vi "test starburst double complete rainbow.vi"() -> ()   [LabVIEW 2015]
uses:
  connection/connection maintainer.lvclass
  client/connection client.lvclass/connection client.ctl
  message/communicator message.lvclass
  starburst/starburst.lvclass
  communicator/communicator.lvclass/communicator.ctl
  message/communicator message.lvclass/communicator message.ctl
  communicator/enqueue variety.ctl
  client/prepare client.vi
  server/prepare server.vi
  TCP client/TCP client.lvclass
  TCP/TCP server.lvclass
  Queue Client/Queue client.lvclass
  communicator/communicator.lvclass
  <vilib>/ptbypt/NI_PtbyPt.lvlib
  manager/queue manager.lvclass
  Queue server/Queue server.lvclass
panel:
  out "ClienQ 2":refnum<class "connection maintainer.lvclass">
  out "Numeric 3":dbl
  out "ClienT 2":timestamp
  out "data 2":variant
  out "ID 2":string
  in  "remake c 2":bool
  in  "c2":cluster{"ID":string, "data":string}
  in  "C to S 2":bool
  out "Numeric 2":dbl
  out "data 3":variant
  out "ID 3":string
  out "data":variant
  out "ID":string
  out "Numeric":dbl
  in  "Boolean":bool
  in  "remake c":bool
  in  "s":cluster{"ID":string, "data":string}
  in  "c1":cluster{"ID":string, "data":string}
  in  "S to C":bool
  in  "C to S":bool
  in  "exits":bool
  out "ClienT":timestamp
  out "servT":timestamp
  out "ClienQ":refnum<class "connection maintainer.lvclass">
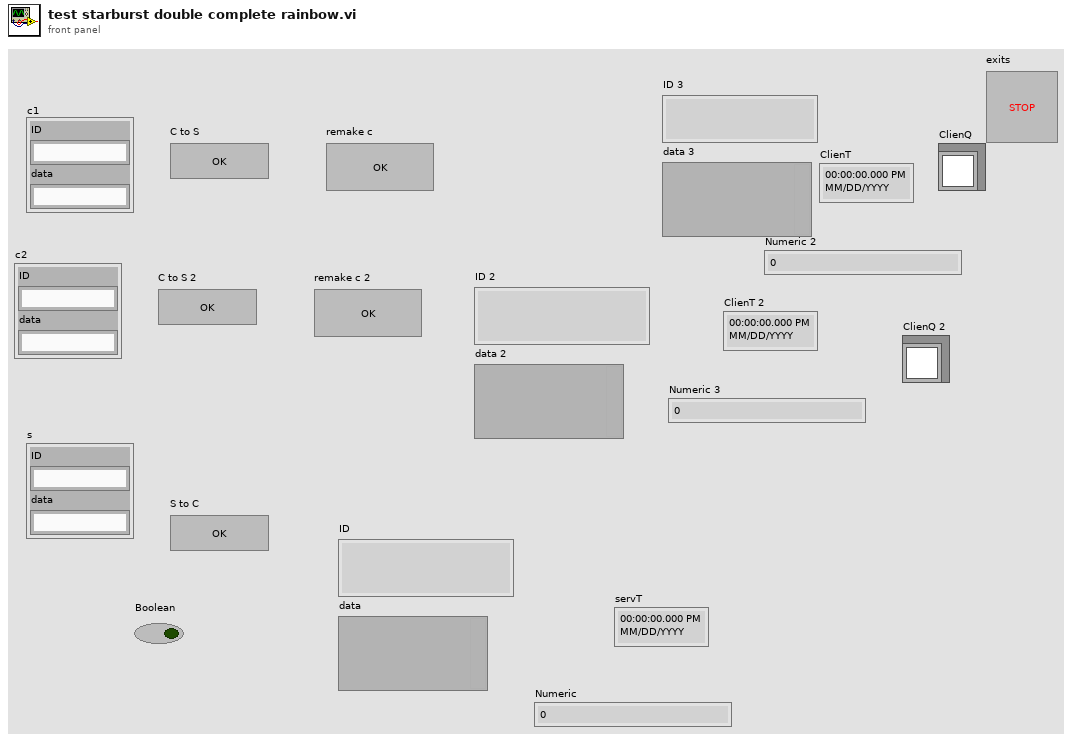
[diagram p1: front panel]
types:
  T1 = typedef "communicator.lvclass/enqueue variety.ctl" = enum16{"normal", "lossy", "priority"}
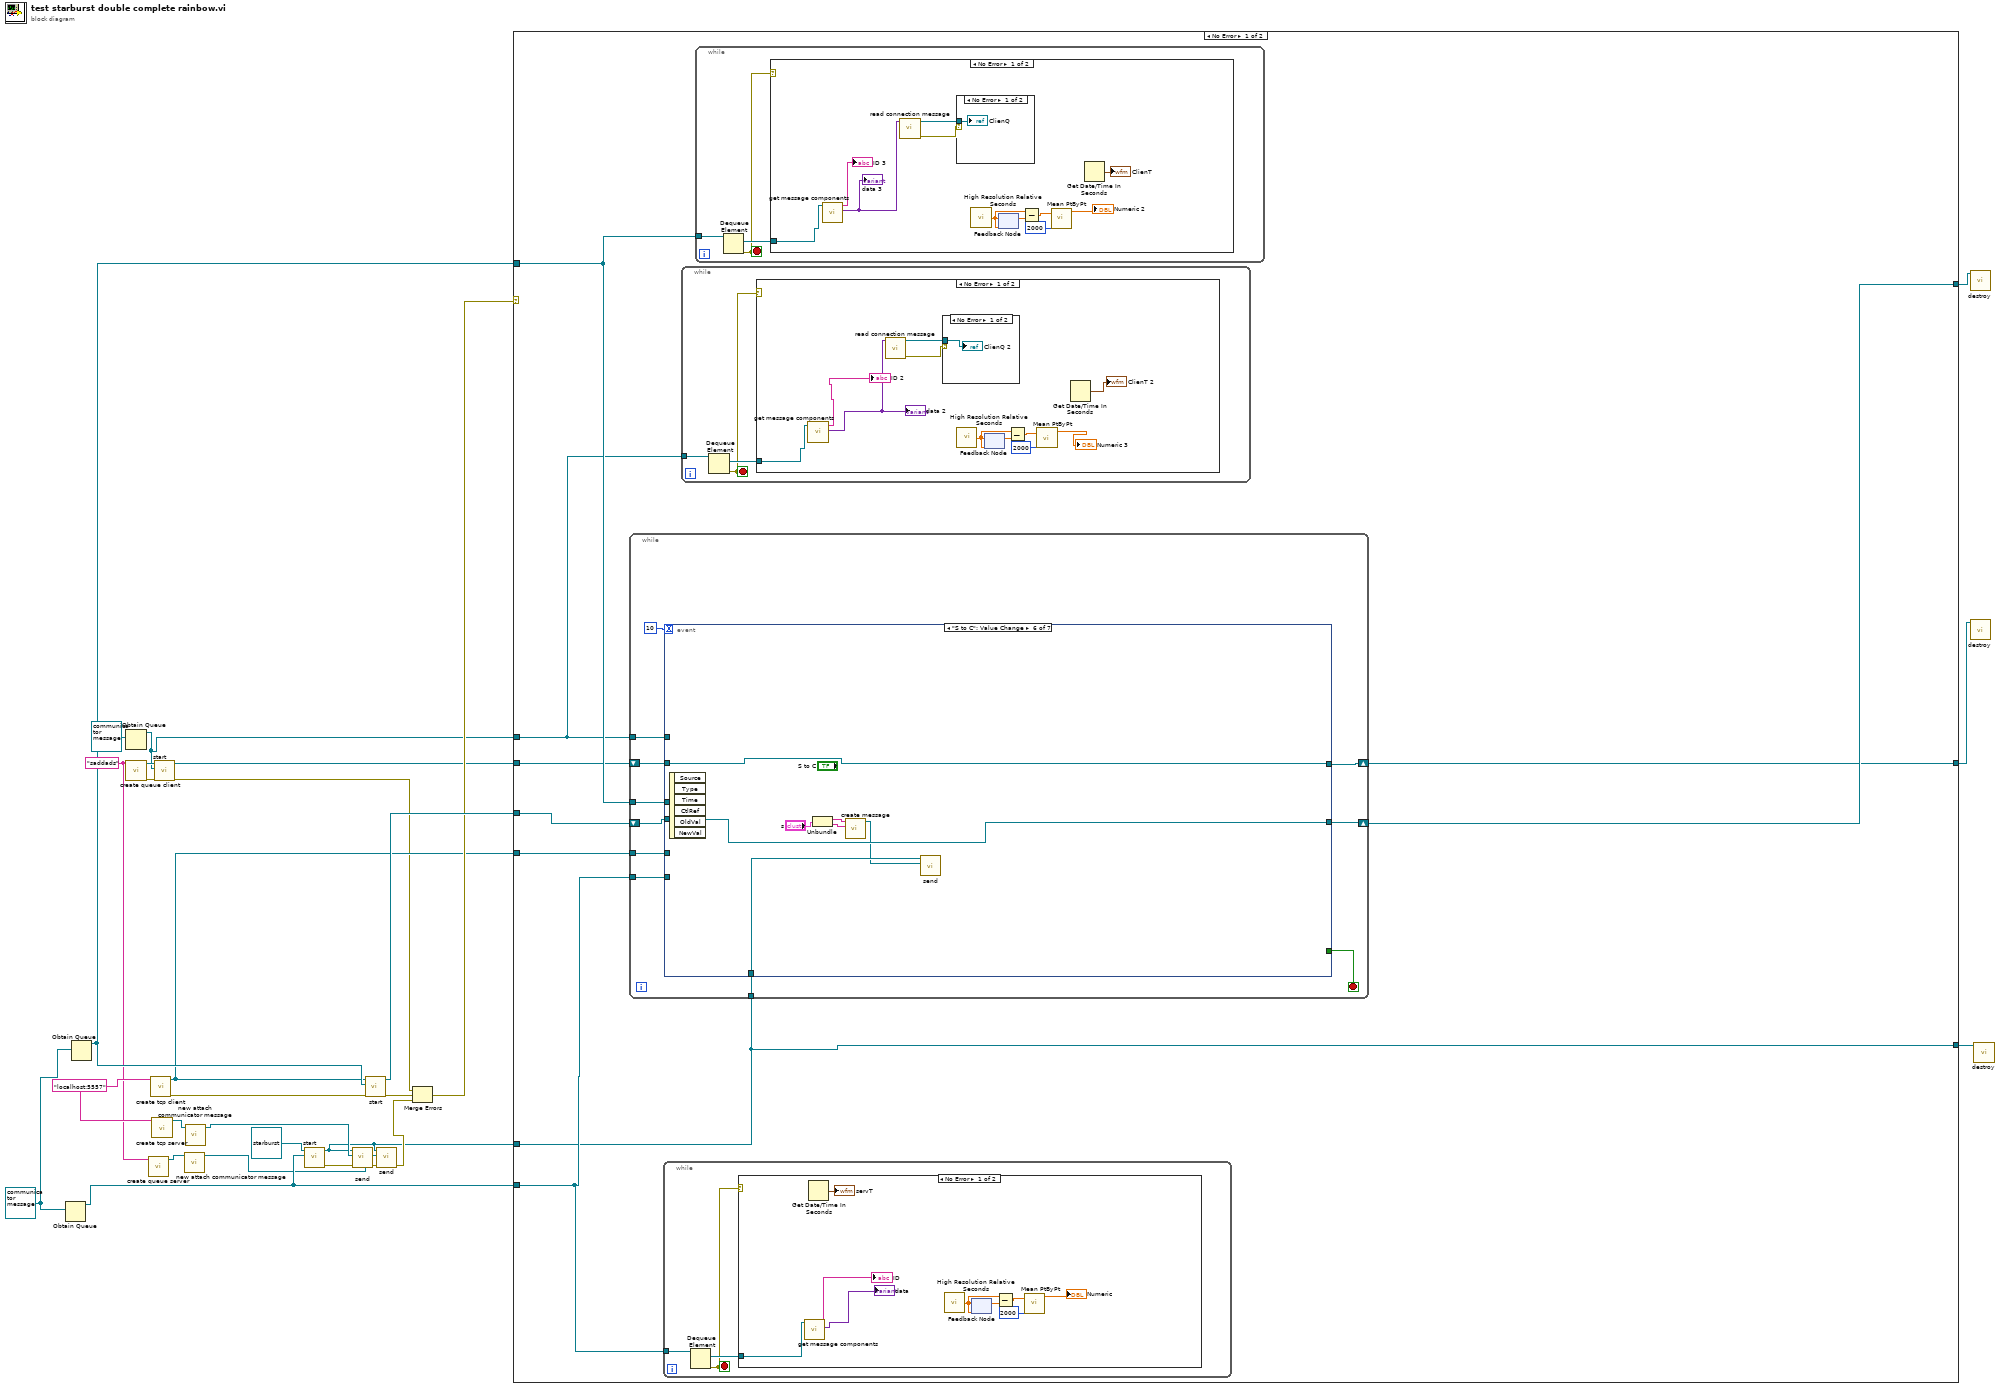
[diagram p0: block diagram]
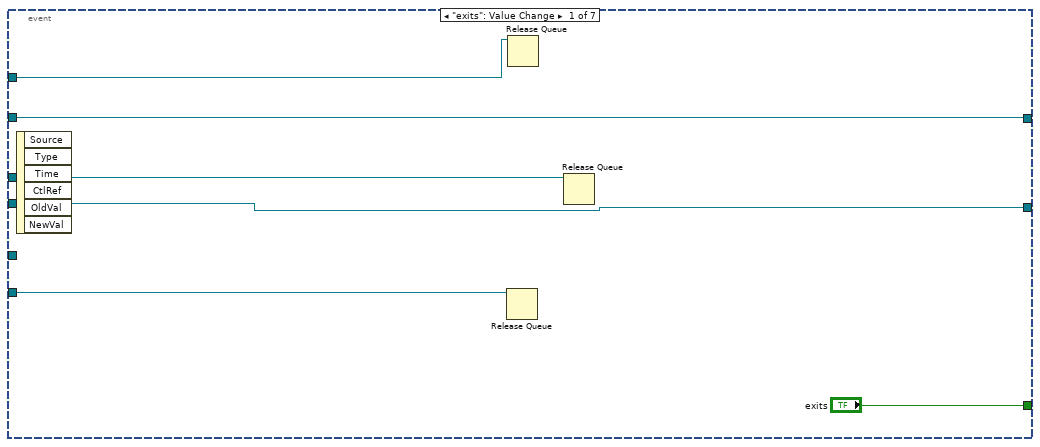
[diagram p4: hidden frame]
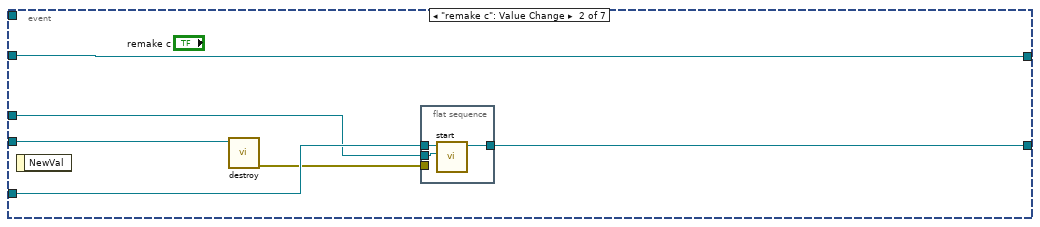
[diagram p5: hidden frame]
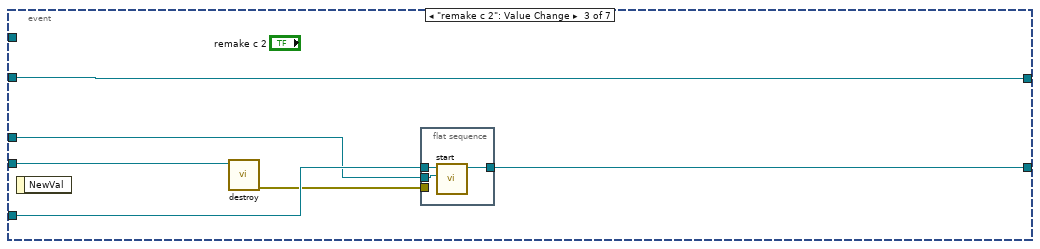
[diagram p6: hidden frame]
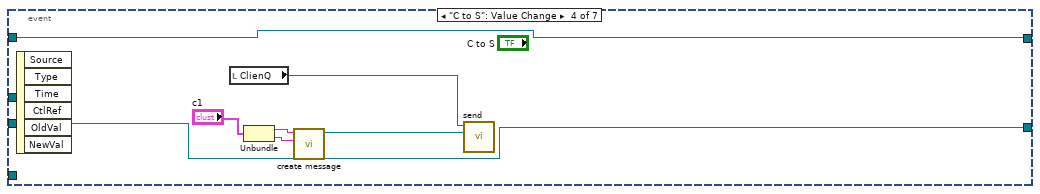
[diagram p7: hidden frame]
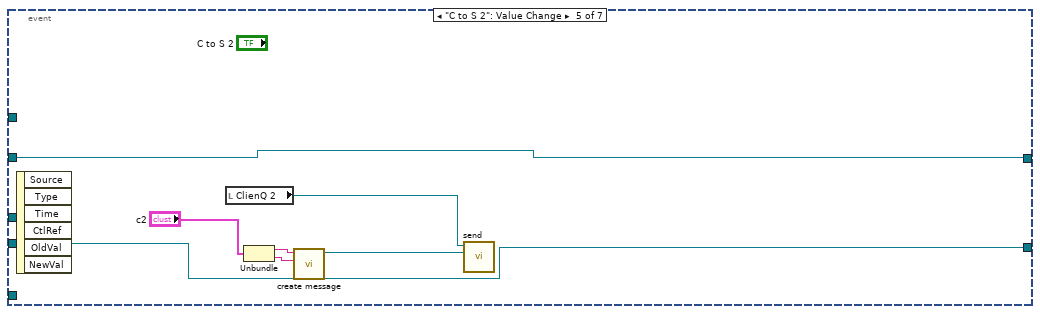
[diagram p8: hidden frame]
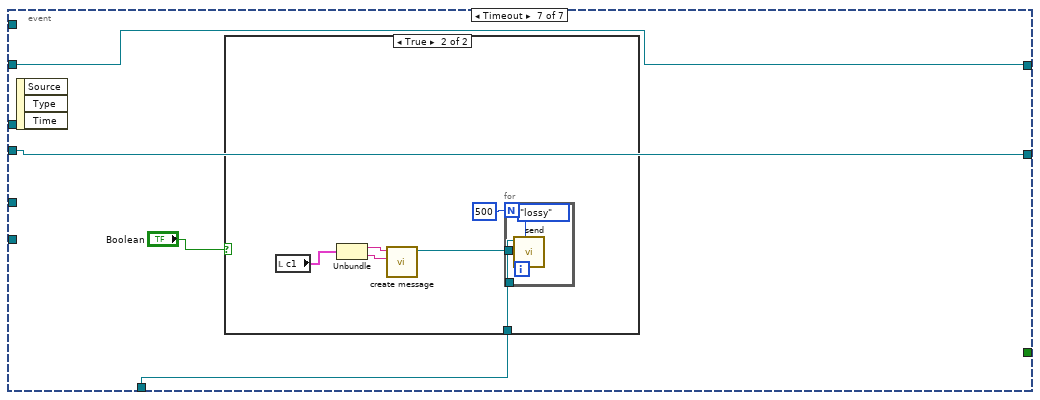
[diagram p9: hidden frame]
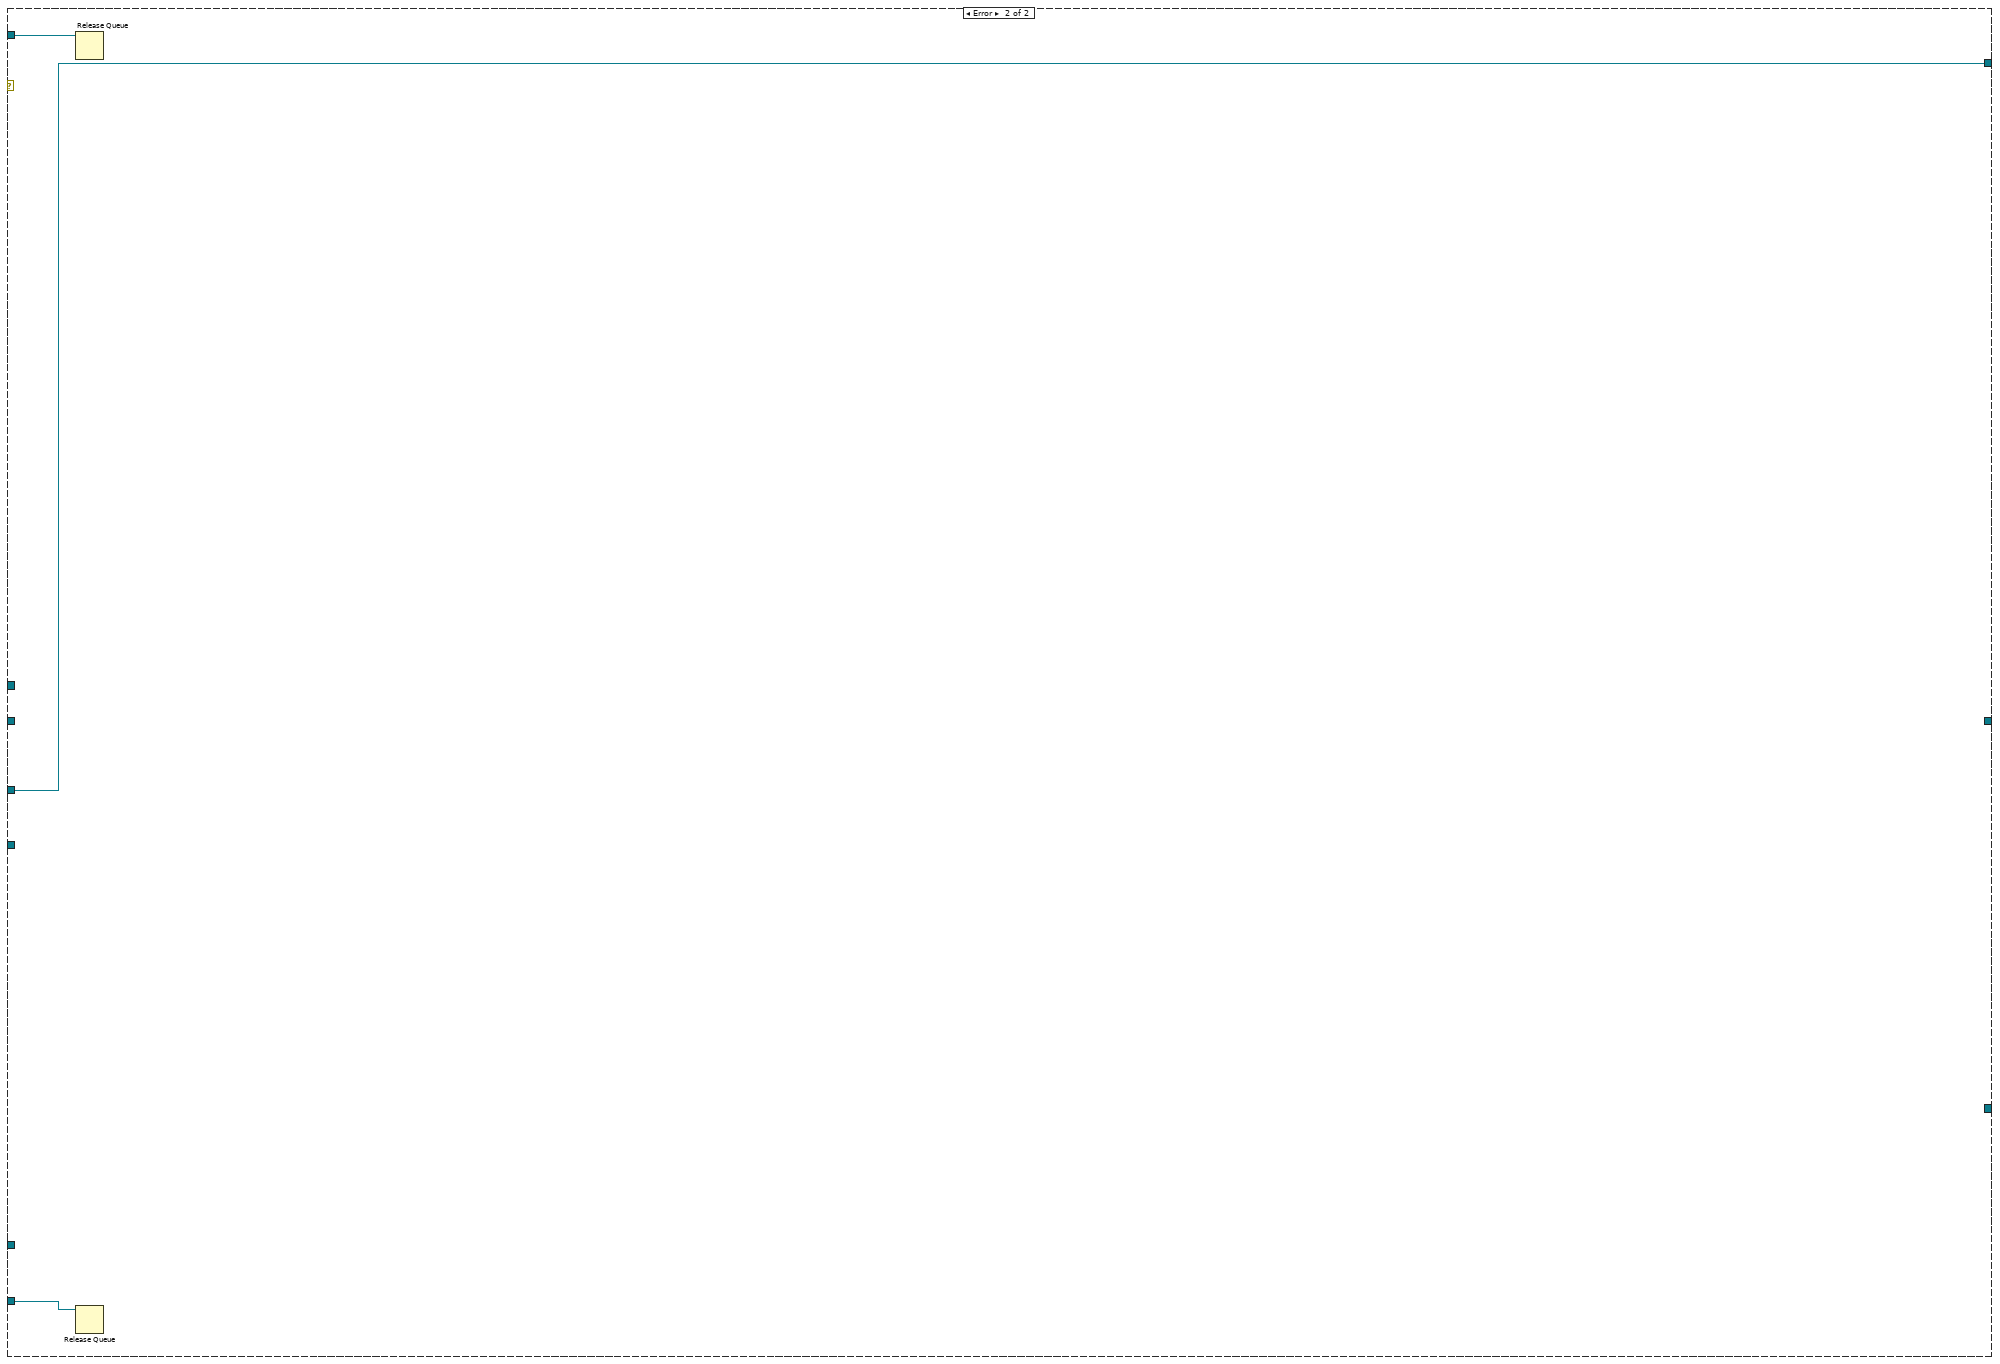
[diagram p14: hidden frame]
diagram:
  w1 = "saddads" ("connection string")
  w20 = refnum<class "communicator message.lvclass"> refnum ("message")
  w24 = "localhost:5557" ("connection string")
  n1 = Obtain Queue(element data type=w20) -> (queue out=w18:refnum<queue>)  [unwired: 4 in, 2 out]
  n2 = Obtain Queue(element data type=w20) -> (queue out=w22:refnum<queue>)  [unwired: 4 in, 2 out]
  n3 = Obtain Queue(element data type=refnum<class "communicator message.lvclass"> refnum ("communicator message.lvclass")) -> (queue out=w3:refnum<queue>)  [unwired: 4 in, 2 out]
  n4 = call "create queue client.vi"("conn string"=w1) -> ("error out"=w6:errorcluster, "TCP client out"=w7:refnum<class "Queue client.lvclass">)  [unwired: 9 in]
  n5 = call "create queue server.vi"("conn string"=w1) -> ("TCP server out"=w12:refnum<class "Queue server.lvclass">)  [unwired: 9 in, 1 out]
  n6 = call "create tcp client.vi"("conn string"=w24) -> ("error out"=w27:errorcluster, "TCP client out"=w21:refnum<class "TCP client.lvclass">)  [unwired: 9 in]
  n7 = call "create tcp server.vi"("conn string"=w24) -> ("TCP server out"=w16:refnum<class "TCP server.lvclass">)  [unwired: 9 in, 1 out]
  n8 = call-dynamic "start.vi"("error in"=w6, "queue to parent"=w3, "communicator in"=w7) -> ("error out"=w5:errorcluster, "communicator out"=w4:refnum<class "Queue client.lvclass">)  [unwired: 7 in]
  n9 = call "new attach communicator message.vi"("comm"=w12) -> ("message"=w9:refnum<class "communicator message.lvclass">)  [unwired: 9 in, 1 out]
  n10 = call "new attach communicator message.vi"("comm"=w16) -> ("message"=w14:refnum<class "communicator message.lvclass">)  [unwired: 9 in, 1 out]
  n11 = call-dynamic "start.vi"("queue to parent"=w18, "communicator in"=refnum<class "starburst.lvclass"> refnum ("starburst")) -> ("error out"=w17:errorcluster, "communicator out"=w10:refnum<class "starburst.lvclass">)  [unwired: 8 in]
  n12 = call "send.vi"("error in"=w17, "element"=w14, "communicator in"=w10) -> ("error out"=w15:errorcluster)  [unwired: 8 in]
  n13 = call-dynamic "start.vi"("error in"=w27, "queue to parent"=w22, "communicator in"=w21) -> ("error out"=w25:errorcluster, "communicator out"=w26:refnum<class "TCP client.lvclass">)  [unwired: 7 in]
  n14 = call "send.vi"("error in"=w15, "element"=w9, "communicator in"=w10) -> ("error out"=w11:errorcluster)  [unwired: 8 in]
  n15 = Merge Errors(w5, w25, w11) -> (w23:errorcluster)
  n16 = case shown="No Error" w23 {
    tunnel: [w33 w150] -> w28
    tunnel: w22 -> [w36 w151]
    tunnel: w26 -> [w35 w150]
    tunnel: w18 -> [w37 w149]
    tunnel: w21 -> [w34 _]
    tunnel: w10 -> [w32 _]
    tunnel: [w32 _] -> w13
    tunnel: w4 -> [w31 _]
    tunnel: w3 -> [w30 _]
    tunnel: [w29 _] -> w2
    frame No Error {
      n17 = while {
        tunnel: w37 -> [w62]
        tunnel: w36 -> [w61]
        tunnel: w34 -> [w59]
        shift-right: [w58] -> w33
        shift-left: w35 -> [w60]
        tunnel: w32 -> [w56]
        shift-right: [w53] -> w29
        shift-left: w31 -> [w55]
        tunnel: w30 -> [w54]
        stop <- w63 stop-if-true
        n18 = event shown="[5] \"S to C\": Value Change" {
          selector: _ -> [_ _ _ _ _ _ _]
          dyn-events: _ -> [_ _ _ _ _ _ _]
          timeout: 10 -> [_ _ _ _ _ _ _]
          tunnel: ["exits" _ _ _ _ _ _] -> w63
          tunnel: w62 -> [w68 _ _ _ _ _ _]
          tunnel: w61 -> [w67 w72 w81 _ _ _ _]
          tunnel: w60 -> [w66 w75 w84 w92 w99 w108 w112]
          tunnel: w59 -> [_ w74 w83 _ _ _ _]
          tunnel: [w66 w71 w80 w92 w99 w108 w112] -> w58
          tunnel: w56 -> [_ _ _ _ _ w104 w110]
          tunnel: w55 -> [w65 w70 w79 w88 w96 w102 w109]
          tunnel: w54 -> [w64 _ _ _ _ _ _]
          tunnel: [w65 w70 w79 w88 w96 w102 w109] -> w53
          event "exits": Value Change {
            n19 = event-data() -> ()  [unwired: 1 in, 6 out]
            n20 = Release Queue(queue=w68) -> ()  [unwired: 2 in, 3 out]
            n21 = Release Queue(queue=w64) -> ()  [unwired: 2 in, 3 out]
            n22 = Release Queue(queue=w67) -> ()  [unwired: 2 in, 3 out]
          }
          event "remake c": Value Change {
            n23 = event-data() -> ()  [unwired: 1 in, 1 out]
            n24 = call-dynamic "destroy.vi"("communicator in"=w75) -> ("error out"=w73:errorcluster)  [unwired: 10 in]
            n25 = flat-sequence {
              tunnel: w74 -> [w78]
              tunnel: w73 -> [_]
              tunnel: w72 -> [w77]
              tunnel: [w76] -> w71
              frame #0 {
                n26 = call-dynamic "start.vi"("queue to parent"=w77, "communicator in"=w78) -> ("communicator out"=w76:refnum<class "TCP client.lvclass">)  [unwired: 8 in, 1 out]
              }
            }
          }
          event "remake c 2": Value Change {
            n27 = event-data() -> ()  [unwired: 1 in, 1 out]
            n28 = call-dynamic "destroy.vi"("communicator in"=w84) -> ("error out"=w82:errorcluster)  [unwired: 10 in]
            n29 = flat-sequence {
              tunnel: w83 -> [w87]
              tunnel: w82 -> [_]
              tunnel: w81 -> [w86]
              tunnel: [w85] -> w80
              frame #0 {
                n30 = call-dynamic "start.vi"("queue to parent"=w86, "communicator in"=w87) -> ("communicator out"=w85:refnum<class "TCP client.lvclass">)  [unwired: 8 in, 1 out]
              }
            }
          }
          event "C to S": Value Change {
            n31 = event-data() -> ()  [unwired: 1 in, 6 out]
            n32 = local read "ClienQ"() -> (w94:refnum<class "connection maintainer.lvclass">)
            n33 = Unbundle("c1") -> ("ID"=w91:string, "data"=w90:string)
            n34 = call "create message.vi"("data"=w90, "ID"=w91) -> ("message"=w93:refnum<class "communicator message.lvclass">)  [unwired: 9 in]
            n35 = call "send.vi"("element"=w93, "communicator in"=w94) -> ()  [unwired: 9 in, 1 out]
          }
          event "C to S 2": Value Change {
            n36 = event-data() -> ()  [unwired: 1 in, 6 out]
            n37 = local read "ClienQ 2"() -> (w101:refnum<class "connection maintainer.lvclass">)
            n38 = Unbundle("c2") -> ("ID"=w98:string, "data"=w97:string)
            n39 = call "create message.vi"("data"=w97, "ID"=w98) -> ("message"=w100:refnum<class "communicator message.lvclass">)  [unwired: 9 in]
            n40 = call "send.vi"("element"=w100, "communicator in"=w101) -> ()  [unwired: 9 in, 1 out]
          }
          event "S to C": Value Change {
            n41 = event-data() -> ()  [unwired: 1 in, 6 out]
            n42 = Unbundle("s") -> ("ID"=w107:string, "data"=w106:string)
            n43 = call "create message.vi"("data"=w106, "ID"=w107) -> ("message"=w103:refnum<class "communicator message.lvclass">)  [unwired: 9 in]
            n44 = call "send.vi"("element"=w103, "communicator in"=w104) -> ()  [unwired: 9 in, 1 out]
          }
          event Timeout {
            n45 = event-data() -> ()  [unwired: 1 in, 3 out]
            n46 = case shown="True" "Boolean" {
              tunnel: w110 -> [_ w114]
              frame False {
              }
              frame True {
                n47 = local read "c1"() -> (w116:cluster{"ID":string, "data":string})
                n48 = Unbundle(w116) -> ("ID"=w118:string, "data"=w117:string)
                n49 = call "create message.vi"("data"=w117, "ID"=w118) -> ("message"=w115:refnum<class "communicator message.lvclass">)  [unwired: 9 in]
                n50 = for {
                  N: 500 -> [_]
                  tunnel: w115 -> [w121]
                  tunnel: w114 -> [w120]
                  n51 = call "send.vi"("enqueue setting"=enqueue_variety."lossy", "element"=w121, "communicator in"=w120) -> ()  [unwired: 8 in, 1 out]
                }
              }
            }
          }
        }
      }
      n52 = while {
        tunnel: w37 -> [w124]
        stop <- w122 stop-if-true
        n53 = Dequeue Element(queue=w124) -> (element=w123:refnum<class "communicator message.lvclass">, error out=w122:errorcluster)  [unwired: 2 in, 2 out]
        n54 = case shown="No Error" w122 {
          tunnel: w123 -> [w125 _]
          frame No Error {
            n55 = call "get message components.vi"("message"=w125) -> ("data"=→"data":variant, "ID"=→"ID":string)  [unwired: 9 in]
            n56 = Get Date/Time In Seconds() -> (seconds since 1Jan1904=→"servT":timestamp)
            n57 = call <vilib>:"High Resolution Relative Seconds.vi"() -> ("relative seconds"=w131:dbl)
            n58 = feedback-in #1(w131) -> ()
            n59 = feedback #1(w131) -> (w132:dbl)
            n60 = Subtract(x=w131, y=w132) -> (x-y=w130:dbl)
            n61 = call <vilib>:"Mean PtByPt.vi"("x"=w130, "sample length"=2000) -> ("mean"=→"Numeric":dbl)  [unwired: 2 in, 1 out]
          }
          frame Error {
          }
        }
      }
      n62 = while {
        tunnel: w30 -> [w40]
        stop <- w38 stop-if-true
        n63 = Dequeue Element(queue=w40) -> (element=w39:refnum<class "communicator message.lvclass">, error out=w38:errorcluster)  [unwired: 2 in, 2 out]
        n64 = case shown="No Error" w38 {
          tunnel: w39 -> [w49 _]
          frame No Error {
            n65 = call "get message components.vi"("message"=w49) -> ("data"=w41:variant, "ID"=→"ID 2":string)  [unwired: 9 in]
            "data 2" <- w41
            n66 = call "read connection message.vi"("data"=w41) -> ("error out"=w50:errorcluster, "conn"=w51:refnum<class "connection maintainer.lvclass">)  [unwired: 9 in]
            n67 = case shown="No Error" w50 {
              tunnel: w51 -> [w52 _]
              frame No Error {
                "ClienQ 2" <- w52
              }
              frame Error {
              }
            }
            n68 = call <vilib>:"High Resolution Relative Seconds.vi"() -> ("relative seconds"=w46:dbl)
            n69 = feedback #2(w46) -> (w45:dbl)
            n70 = feedback-in #2(w46) -> ()
            n71 = Subtract(x=w46, y=w45) -> (x-y=w47:dbl)
            n72 = call <vilib>:"Mean PtByPt.vi"("x"=w47, "sample length"=2000) -> ("mean"=→"Numeric 3":dbl)  [unwired: 2 in, 1 out]
            n73 = Get Date/Time In Seconds() -> (seconds since 1Jan1904=→"ClienT 2":timestamp)
          }
          frame Error {
          }
        }
      }
      n74 = while {
        tunnel: w36 -> [w136]
        stop <- w134 stop-if-true
        n75 = Dequeue Element(queue=w136) -> (element=w135:refnum<class "communicator message.lvclass">, error out=w134:errorcluster)  [unwired: 2 in, 2 out]
        n76 = case shown="No Error" w134 {
          tunnel: w135 -> [w143 _]
          frame No Error {
            n77 = call "get message components.vi"("message"=w143) -> ("data"=w142:variant, "ID"=→"ID 3":string)  [unwired: 9 in]
            "data 3" <- w142
            n78 = call "read connection message.vi"("data"=w142) -> ("error out"=w146:errorcluster, "conn"=w147:refnum<class "connection maintainer.lvclass">)  [unwired: 9 in]
            n79 = case shown="No Error" w146 {
              tunnel: w147 -> [w148 _]
              frame No Error {
                "ClienQ" <- w148
              }
              frame Error {
              }
            }
            n80 = call <vilib>:"High Resolution Relative Seconds.vi"() -> ("relative seconds"=w138:dbl)
            n81 = feedback #3(w138) -> (w137:dbl)
            n82 = feedback-in #3(w138) -> ()
            n83 = Subtract(x=w138, y=w137) -> (x-y=w139:dbl)
            n84 = call <vilib>:"Mean PtByPt.vi"("x"=w139, "sample length"=2000) -> ("mean"=→"Numeric 2":dbl)  [unwired: 2 in, 1 out]
            n85 = Get Date/Time In Seconds() -> (seconds since 1Jan1904=→"ClienT":timestamp)
          }
          frame Error {
          }
        }
      }
    }
    frame Error {
      n86 = Release Queue(queue=w151) -> ()  [unwired: 2 in, 3 out]
      n87 = Release Queue(queue=w149) -> ()  [unwired: 2 in, 3 out]
    }
  }
  n88 = call-dynamic "destroy.vi"("communicator in"=w28) -> ()  [unwired: 10 in, 1 out]
  n89 = call-dynamic "destroy.vi"("communicator in"=w2) -> ()  [unwired: 10 in, 1 out]
  n90 = call-dynamic "destroy.vi"("communicator in"=w13) -> ()  [unwired: 10 in, 1 out]
